vi "Get Arg Map.vi"(8 "error in (no error)":errorcluster, 11 "Arguments in":refnum<class "Values.lvclass">) -> (0 "error out":errorcluster, 2 "Arguments":map{string, variant}(c390), 3 "Arguments out":refnum<class "Values.lvclass">)   [LabVIEW 2020, in "HTTP Server.lvlib" / "Values.lvclass"]
uses:
  Values.lvclass
  Values.lvclass/Values.ctl
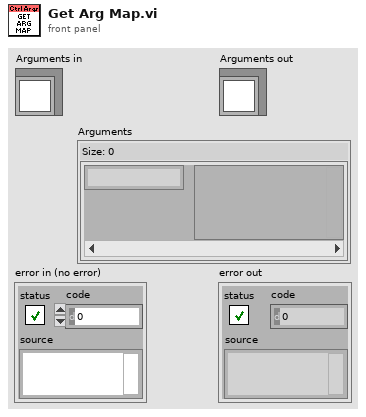
[diagram p1: front panel]
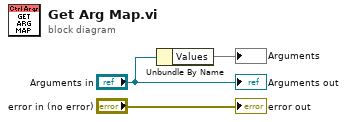
[diagram p0: block diagram]
diagram:
  n1 = Unbundle By Name("Arguments in") -> ("Values"=→"Arguments":map{string, variant})
  "error out" <- "error in (no error)"
  "Arguments out" <- "Arguments in"
